vi "InitializeMain.vi"(8 "error in":errorcluster, 11 "Inputs In":T1={"File Name"="", "Force (Hz)"=0.0, "Camera (Hz)"=0.0, "Systole (V)"=0.0, "Diastole (V)"=0.0, "T (sec)"=0.0, "Delay (sec)"=0.0, "Setpoint Function"=enum."Incremental PWM Step", "Max Diam (mm)"=0.0, "DAQmx Servo Task"="MyPulseOutputTask", "Force Sensor Channel"="Dev2/ai7", "DAQmx LED Task"="MyDigitalOutTask", "Camera Selector"="cam5", "FS Task Out"="", "Servo Task Out"="", "LED Task Out"="", "Camera Session Out"="", "Color Pane"=0} {"Color Pane" items=["Blue", "Red", "Green", "Saturation", "Value", "Intensity", "Luminance", "Hue", ""]}) -> (0 "error out":errorcluster, 1 "New Image":T4, 3 "Inputs Out":T1={"File Name"="", "Force (Hz)"=0.0, "Camera (Hz)"=0.0, "Systole (V)"=0.0, "Diastole (V)"=0.0, "T (sec)"=0.0, "Delay (sec)"=0.0, "Setpoint Function"=enum."Incremental PWM Step", "Max Diam (mm)"=0.0, "DAQmx Servo Task"="MyPulseOutputTask", "Force Sensor Channel"="Dev2/ai7", "DAQmx LED Task"="MyDigitalOutTask", "Camera Selector"="cam5", "FS Task Out"="", "Servo Task Out"="", "LED Task Out"="", "Camera Session Out"="", "Color Pane"=0} {"Color Pane" items=["Blue", "Red", "Green", "Saturation", "Value", "Intensity", "Luminance", "Hue", ""]}, 5 "Start Time":timestamp)   [LabVIEW 2020]
uses:
  Controls/Inputs.ctl
  Controls/Serpoint.ctl
  <vilib>/userDefined/High Color/IMAQdx.ctl
  <vilib>/vision/Image Controls.llb/IMAQ Image.ctl
  <vilib>/DAQmx/create/channels.llb/DAQmx Create Channel (AI-Voltage-Basic).vi
  <vilib>/DAQmx/configure/timing.llb/DAQmx Timing (Sample Clock).vi
  <vilib>/vision/driver/NI_Vision_Acquisition_Software.lvlib
panel:
  # "Test Variables:"
  # "Sampling Frequencies:"
  # "Test Variables:"
  # "Sampling Frequencies:"
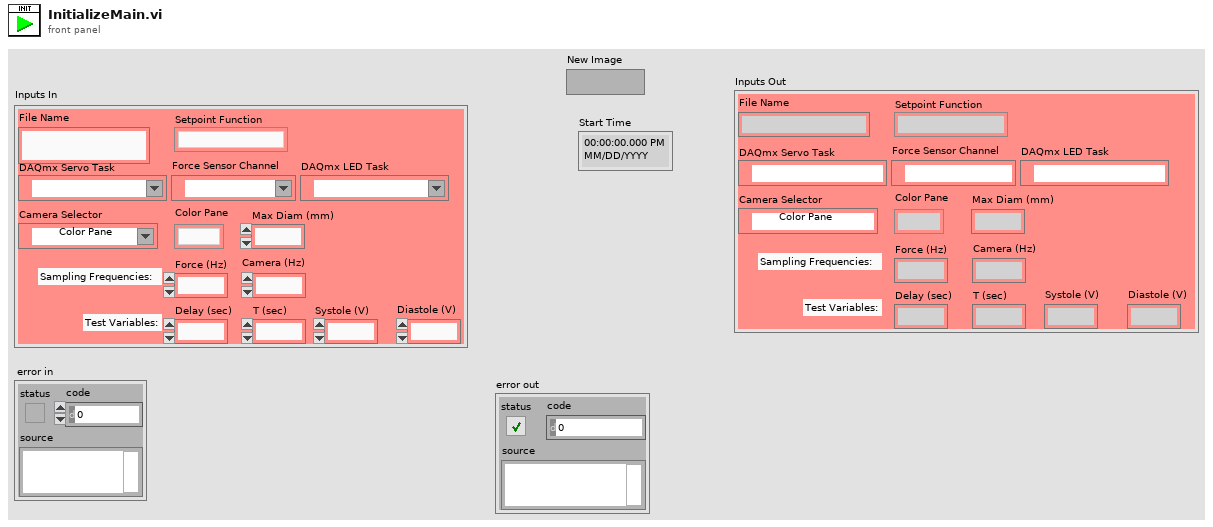
[diagram p1: front panel]
types:
  T1 = typedef "Inputs.ctl" = cluster{"File Name":string, "Force (Hz)":dbl, "Camera (Hz)":dbl, "Systole (V)":dbl, "Diastole (V)":dbl, "T (sec)":dbl, "Delay (sec)":dbl, "Setpoint Function":T2, "Max Diam (mm)":dbl, "DAQmx Servo Task":refnum<k21>, "Force Sensor Channel":tag, "DAQmx LED Task":refnum<k21>, "Camera Selector":T3, "FS Task Out":refnum<k21>, "Servo Task Out":refnum<k21>, "LED Task Out":refnum<k21>, "Camera Session Out":T3, "Color Pane":i32}
  T2 = typedef "Serpoint.ctl" = enum16{"Incremental PWM Step", "PWM Step", "Ramp", "Sinusoidal", "Blood-Pressure"}
  T3 = typedef "IMAQdx.ctl" = refnum<k21>
  T4 = typedef "IMAQ Image.ctl" = refnum<image>
  T5 = typedef "Image Type" = u32
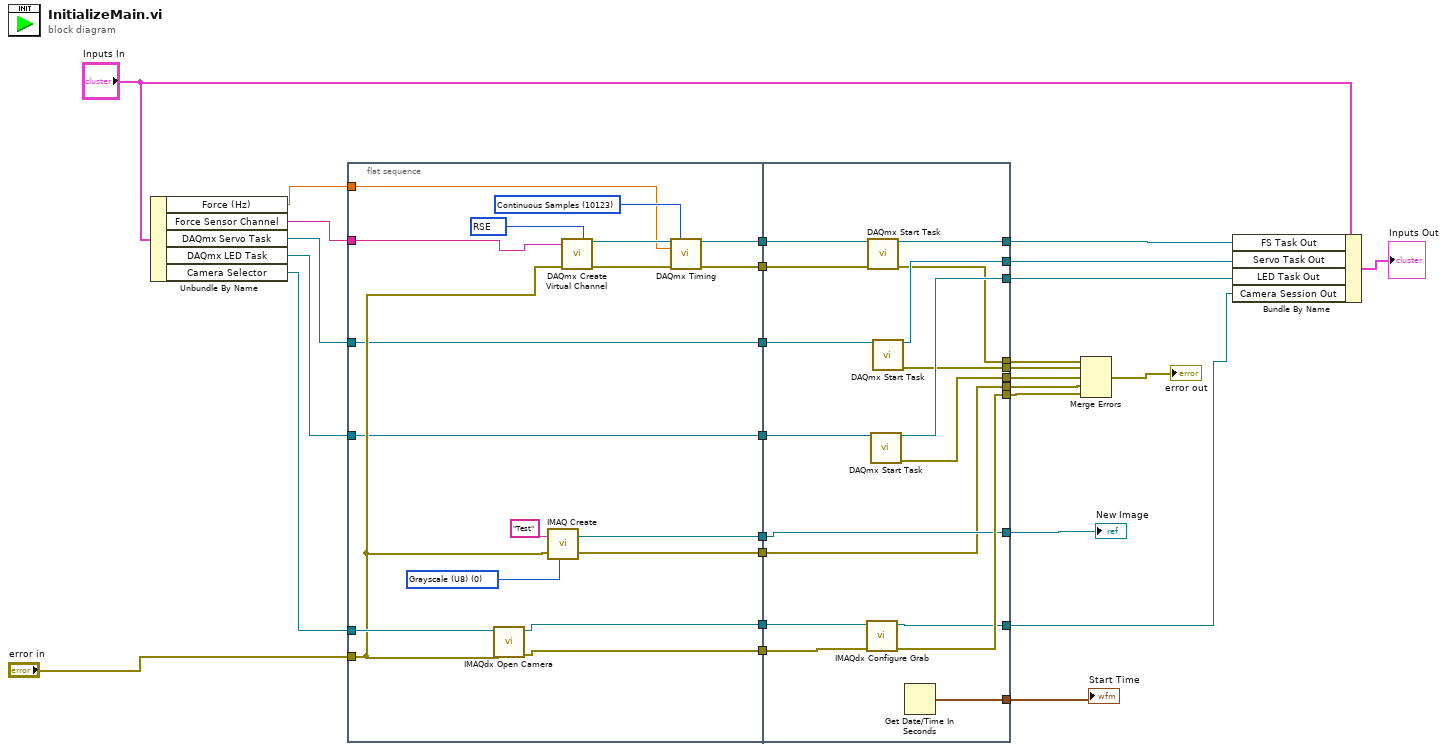
[diagram p0: block diagram]
diagram:
  n1 = Unbundle By Name("Inputs In") -> ("Force (Hz)"=w24:dbl, "Force Sensor Channel"=w10:tag, "DAQmx Servo Task"=w9:refnum<k21>, "DAQmx LED Task"=w8:refnum<k21>, "Camera Selector"=w2:T3)
  n2 = flat-sequence {
    tunnel: w2 -> [w40]
    tunnel: [w39] -> w28
    tunnel: [w38] -> w27
    tunnel: [w37] -> w26
    tunnel: [w36] -> w25
    tunnel: w24 -> [w35]
    tunnel: "error in" -> [w33]
    tunnel: [w34] -> w18
    tunnel: [w32] -> w15
    tunnel: [w30] -> w12
    tunnel: [w29] -> w11
    tunnel: w10 -> [w31]
    tunnel: w9 -> [w30]
    tunnel: w8 -> [w29]
    tunnel: w28 -> [w63]
    tunnel: w27 -> [w62]
    tunnel: w26 -> [w61]
    tunnel: w25 -> [w60]
    tunnel: [w59] -> w6
    tunnel: [w58] -> w5
    tunnel: [w57] -> w4
    tunnel: [w56] -> w22
    tunnel: [w55] -> w21
    tunnel: [w54] -> w20
    tunnel: [w53] -> w16
    tunnel: [w52] -> w1
    tunnel: w18 -> [w51]
    tunnel: [w51] -> w17
    tunnel: w15 -> [w50]
    tunnel: [w50] -> w14
    tunnel: [w49] -> w13
    tunnel: w12 -> [w48]
    tunnel: w11 -> [w47]
    frame #0 {
      w41 = T5 0 items=["Grayscale (U8)", "Grayscale (I16)", "Grayscale (SGL)", "Complex (CSG)", "RGB (U32)", "HSL (U32)", "RGB (U64)", "Grayscale (U16)"] ("Image Type")
      w44 = 10083 items=["Default"=-1, "RSE"=10083, "NRSE"=10078, "Differential"=10106, "Pseudodifferential"=12529] ("input terminal configuration")
      w43 = 10123 items=["Finite Samples"=10178, "Continuous Samples"=10123, "Hardware Timed Single Point"=12522] ("sample mode")
      n3 = call <vilib>:"IMAQdx Open Camera.vi"("error in"=w33, "Session In"=w40) -> ("error out"=w39:errorcluster, "Session Out"=w38:T3)  [unwired: 8 in]
      n4 = call "IMAQ Create"("Image Name"="Test", "Image Type"=w41, "error in (no error)"=w33) -> ("New Image"=w34:T4, "error out"=w32:errorcluster)  [unwired: 2 in]
      n5 = call-poly <vilib>:"DAQmx Create Virtual Channel.vi"("input terminal configuration"=w44, "physical channels"=w31, "error in"=w33) -> ("task out"=w45:refnum<k21>, "error out"=w46:errorcluster)  [unwired: 11 in]
      n6 = call-poly <vilib>:"DAQmx Timing.vi"("task/channels in"=w45, "sample mode"=w43, "rate"=w35, "error in"=w46) -> ("task out"=w37:refnum<k21>, "error out"=w36:errorcluster)  [unwired: 10 in]
    }
    frame #1 {
      n7 = call <vilib>:"IMAQdx Configure Grab.vi"("error in"=w63, "Session In"=w62) -> ("error out"=w53:errorcluster, "Session Out"=w52:T3)  [unwired: 8 in]
      n8 = call <vilib>:"DAQmx Start Task.vi"("task/channels in"=w61, "error in"=w60) -> ("task out"=w59:refnum<k21>, "error out"=w56:errorcluster)  [unwired: 12 in]
      n9 = call <vilib>:"DAQmx Start Task.vi"("task/channels in"=w47) -> ("task out"=w57:refnum<k21>, "error out"=w54:errorcluster)  [unwired: 13 in]
      n10 = call <vilib>:"DAQmx Start Task.vi"("task/channels in"=w48) -> ("task out"=w58:refnum<k21>, "error out"=w55:errorcluster)  [unwired: 13 in]
      n11 = Get Date/Time In Seconds() -> (seconds since 1Jan1904=w49:timestamp)
    }
  }
  n12 = Merge Errors(w22, w21, w20, w14, w16) -> (→"error out":errorcluster)
  n13 = Bundle By Name(cluster="Inputs In", "FS Task Out"=w6, "Servo Task Out"=w5, "LED Task Out"=w4, "Camera Session Out"=w1) -> (→"Inputs Out":T1)
  "New Image" <- w17
  "Start Time" <- w13
